vi "CreateFForVolt (SubVI).vi"(8 "WaitSignalGen":u32=150, 9 "Frequency 1,kHz":dbl, 10 "dFreq, kHz":dbl, 11 "Frequency 2,kHz":dbl) -> (3 "AllParametrArray":dbl[][](array[numeric]))   [LabVIEW 2017]
uses:
  st_voltmetr-master/subVIs/st_str Global.vi
panel:
  out "V":dbl[](array[numeric])
  out "ChangeGenParam":bool
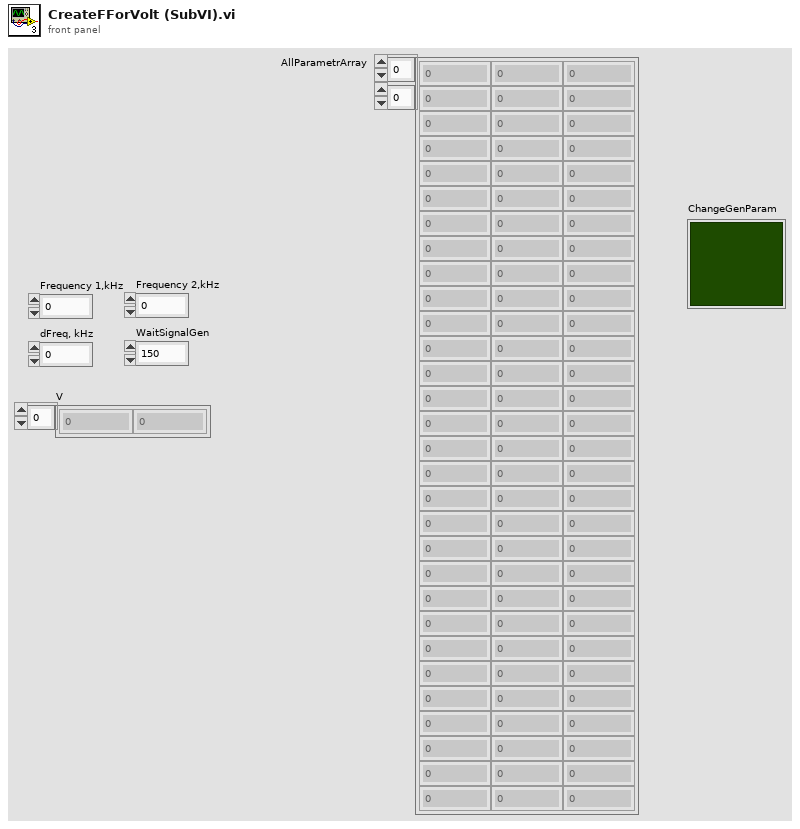
[diagram p1: front panel]
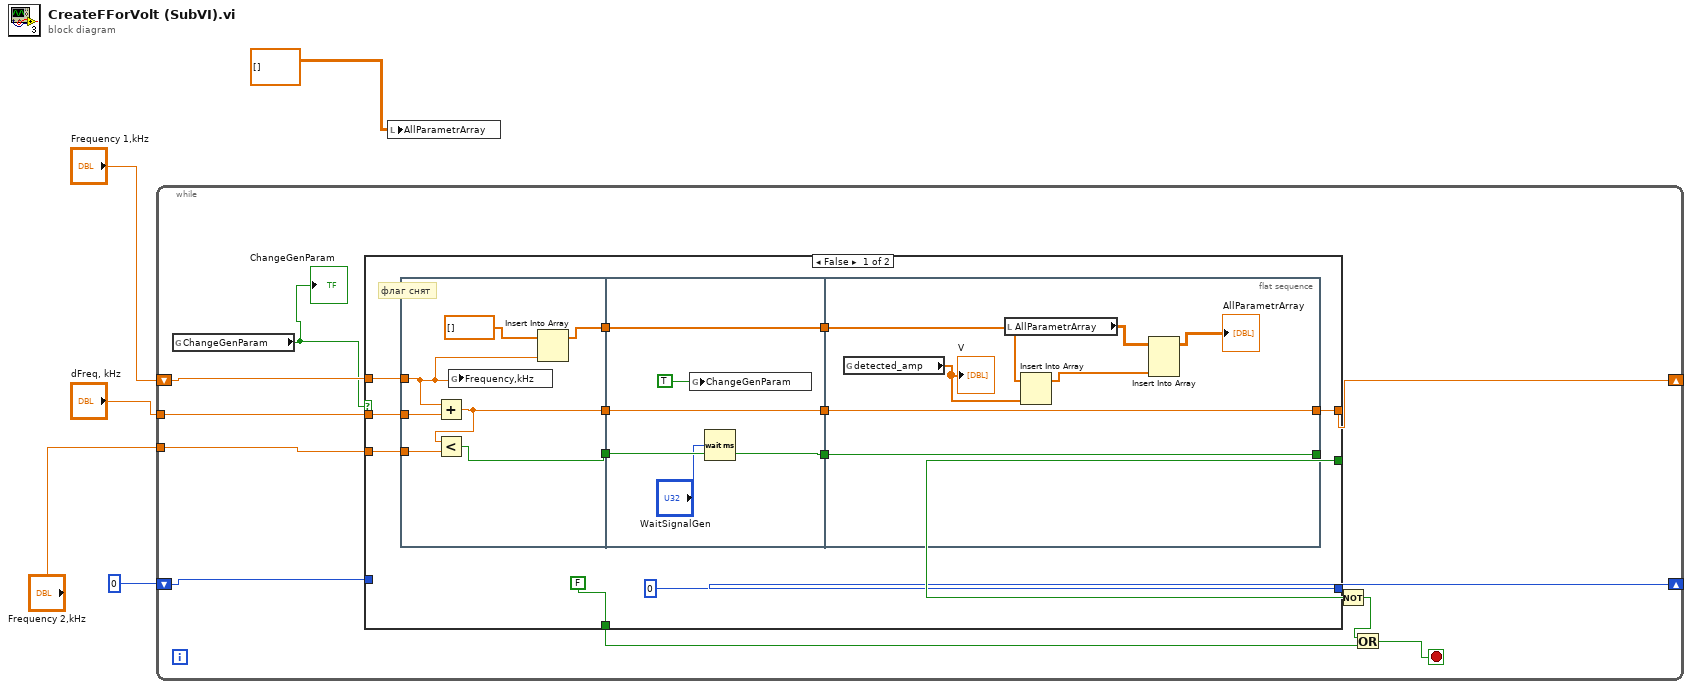
[diagram p0: block diagram]
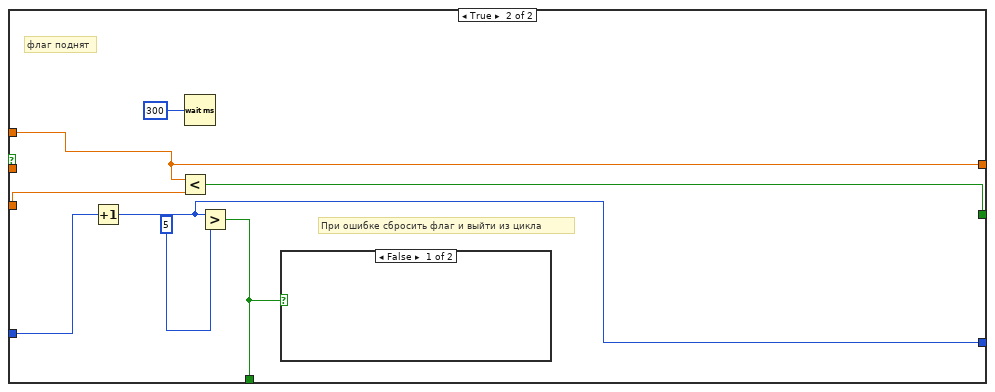
[diagram p2: hidden frame]
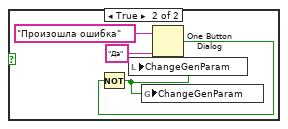
[diagram p3: hidden frame]
diagram:
  n1 = while {
    shift-right: [w15] -> _
    shift-left: "Frequency 1,kHz" -> [w13]
    tunnel: "dFreq, kHz" -> [w16]
    tunnel: "Frequency 2,kHz" -> [w14]
    shift-right: [w8] -> _
    shift-left: 0 -> [w11]
    stop <- w7 stop-if-true
    n2 = global read "st_str Global.vi" "ChangeGenParam"() -> (w6:bool)
    "ChangeGenParam" <- w6
    n3 = case shown="False" w6 {
      tunnel: w16 -> [w29 _]
      tunnel: [w28 w56] -> w15
      tunnel: w14 -> [w27 w55]
      tunnel: [w26 w54] -> w12
      tunnel: w13 -> [w25 w56]
      tunnel: w11 -> [_ w52]
      tunnel: [FALSE w49] -> w9
      tunnel: [0 w50] -> w8
      frame False {
        # "флаг снят"
        n4 = flat-sequence {
          tunnel: w29 -> [w36]
          tunnel: w27 -> [w34]
          tunnel: w25 -> [w31]
          tunnel: [w35] -> w22
          tunnel: [w33] -> w21
          tunnel: [w30] -> w17
          tunnel: w22 -> [w41]
          tunnel: w21 -> [w40]
          tunnel: [w41] -> w20
          tunnel: [w40] -> w19
          tunnel: [w38] -> w18
          tunnel: w17 -> [w38]
          tunnel: [w47] -> w26
          tunnel: [w48] -> w28
          tunnel: w20 -> [w48]
          tunnel: w19 -> [w47]
          tunnel: w18 -> [w45]
          frame #0 {
            n5 = Add(x=w31, y=w36) -> (x+y=w35:dbl)
            n6 = Less?(x=w35, y=w34) -> (x < y?=w33:bool)
            n7 = global write "st_str Global.vi" "Frequency,kHz"(w31) -> ()
            n8 = Insert Into Array(array=dbl[] [], new element=w31) -> (w30:dbl[])  [unwired: 1 in]
          }
          frame #1 {
            n9 = global write "st_str Global.vi" "ChangeGenParam"(TRUE ("ChangeGenParam")) -> ()
            n10 = Wait (ms)(milliseconds to wait="WaitSignalGen") -> ()  [unwired: 1 out]
          }
          frame #2 {
            n11 = global read "st_str Global.vi" "detected_amp"() -> (w46:dbl[])
            "V" <- w46
            n12 = local read "AllParametrArray"() -> (w42:dbl[][])
            n13 = Insert Into Array(array=w45, new element=w46) -> (w44:dbl[])  [unwired: 1 in]
            n14 = Insert Into Array(array=w42, new element=w44) -> (→"AllParametrArray":dbl[][])  [unwired: 2 in]
          }
        }
      }
      frame True {
        # "флаг поднят"
        # "При ошибке сбросить флаг и выйти из цикла"
        n15 = Increment(x=w52) -> (x+1=w50:i32)
        n16 = Less?(x=w56, y=w55) -> (x < y?=w54:bool)
        n17 = Wait (ms)(milliseconds to wait=u32 300) -> ()  [unwired: 1 out]
        n18 = Greater?(x=w50, y=5) -> (0:w49:bool)
        n19 = case shown="False" w49 {
          frame False {
          }
          frame True {
            n20 = One Button Dialog(message="Произошла ошибка", button name ("OK")="Да") -> (true=w57:bool)
            n21 = Not(x=w57) -> (.not. x?=w58:bool)
            n22 = local write "ChangeGenParam"(w58) -> ()
            n23 = global write "st_str Global.vi" "ChangeGenParam"(w58) -> ()
          }
        }
      }
    }
    n24 = Not(x=w12) -> (.not. x?=w10:bool)
    n25 = Or(x=w10, y=w9) -> (x .or. y?=w7:bool)
  }
  n26 = local write "AllParametrArray"(dbl[][] []) -> ()
